vi "(SubVI)Scope_Offset Calibration.vi"(8 "error in (no error)":errorcluster caption="에러 입력(에러 없음)") -> (0 "error out":errorcluster caption="에러 출력")   [LabVIEW 2020]
uses:
  Serial/Controls/(Ctrl)Serial_Write Read Option.ctl
  Serial/Instance VIs/(SubVI)Serial_Write-Read.vi
panel:
  out "Read Data":u8[](array[numeric]) format="%.0x"
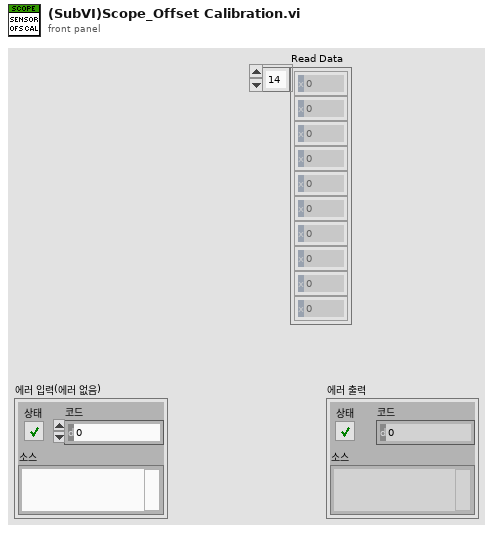
[diagram p1: front panel]
types:
  T1 = typedef "(Ctrl)Serial_Write Read Option.ctl" = cluster{"Echo Request":bool, "Header Verification":bool, "Checksum Verification":bool, "User Code Verifiaction":bool}
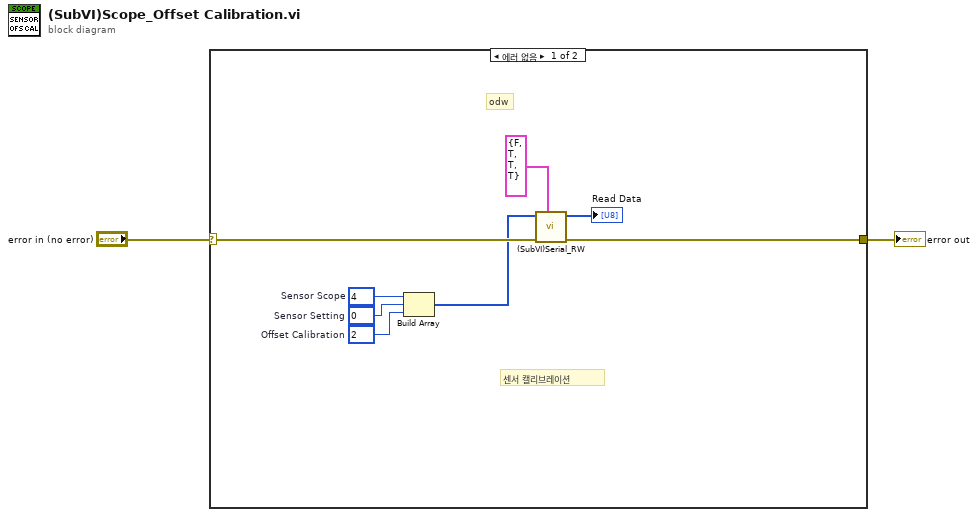
[diagram p0: block diagram]
diagram:
  n1 = case shown="에러 없음" "error in (no error)" {
    selector: "error in (no error)" -> [w8 w11]
    tunnel: [w6 w11] -> w2
    frame No Error {
      w5 = u8 0  # Sensor Setting
      w9 = u8 2  # Offset Calibration
      w10 = u8 4  # Sensor Scope
      # "odw"
      # "센서 캘리브레이션"
      n2 = Build Array(w10, w5, w9) -> (w7:u8[])
      n3 = call-poly "(SubVI)Serial_RW.vi"("Option"=T1 {"Echo Request"=FALSE, "Header Verification"=TRUE, "Checksum Verification"=TRUE, "User Code Verifiaction"=TRUE}, "error in (no error)"=w8, "Data to Write"=w7) -> ("error out"=w6:errorcluster, "Read Data"=→"Read Data":u8[])  [unwired: 6 in, 1 out]
    }
    frame Error {
    }
  }
  "error out" <- w2
